vi "Parse-Most_Common_Tile.vi"(10 "Array":T1[](array[typedef])) -> (2 "Tile":T1)   [LabVIEW 2020]
doc: "<B>Description:</B> takes an array of tiles and determines which is the most common and returns that.\n\n<B>Date:</B> 05/2019\n<B>Author:</B> Luke Jarocki, Choose Movement Consulting, LLC"
uses:
  Controls/TileColor.ctl
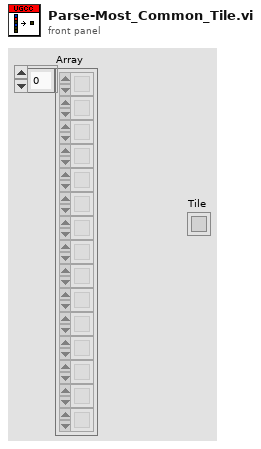
[diagram p1: front panel]
types:
  T1 = typedef "TileColor.ctl" = u16
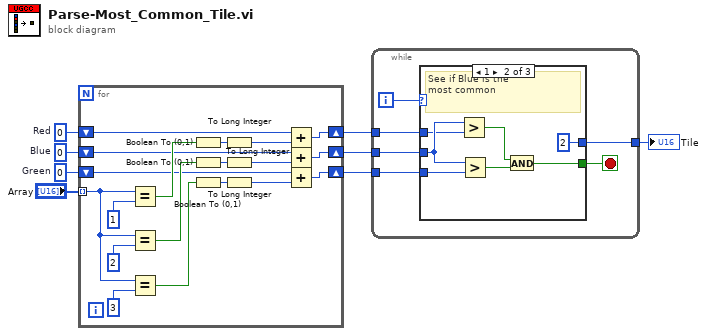
[diagram p0: block diagram]
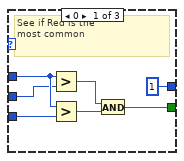
[diagram p2: hidden frame]
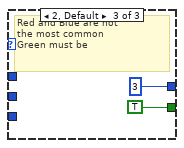
[diagram p3: hidden frame]
diagram:
  w5 = 0  # Green
  w6 = 0  # Blue
  w7 = 0  # Red
  n1 = for {
    tunnel: "Array" -> [w18] mode=indexing
    shift-right: [w24] -> w4
    shift-left: w7 -> [w25]
    shift-right: [w19] -> w3
    shift-left: w6 -> [w20]
    shift-right: [w15] -> w2
    shift-left: w5 -> [w16]
    n2 = Equal?(x=w18, y=T1 1 ("Tile")) -> (x = y?=w26:bool)
    n3 = Equal?(x=w18, y=T1 2 ("Tile")) -> (x = y?=w23:bool)
    n4 = Equal?(x=w18, y=T1 3 ("Tile")) -> (x = y?=w22:bool)
    n5 = Boolean To (0,1)(Boolean=w26) -> (0, 1=w14:i16)
    n6 = Boolean To (0,1)(Boolean=w23) -> (0, 1=w11:i16)
    n7 = Boolean To (0,1)(Boolean=w22) -> (0, 1=w12:i16)
    n8 = To Long Integer(number=w14) -> (32bit integer=w13:i32)
    n9 = To Long Integer(number=w11) -> (32bit integer=w10:i32)
    n10 = To Long Integer(number=w12) -> (32bit integer=w9:i32)
    n11 = Add(x=w25, y=w13) -> (x+y=w24:i32)
    n12 = Add(x=w20, y=w10) -> (x+y=w19:i32)
    n13 = Add(x=w16, y=w9) -> (x+y=w15:i32)
  }
  n14 = while {
    tunnel: w4 -> [w32]
    tunnel: w3 -> [w31]
    tunnel: w2 -> [w30]
    tunnel: [w28] -> w1
    i -> [w33]
    stop <- w29 stop-if-true
    n15 = case shown="1" w33 {
      tunnel: w32 -> [w40 w43 _]
      tunnel: w31 -> [w39 w45 _]
      tunnel: w30 -> [w38 w44 _]
      tunnel: [w35 w42 TRUE] -> w29
      tunnel: [T1 1 ("Tile") T1 2 ("Tile") T1 3 ("Tile")] -> w28
      frame 0 {
        # "See if Red is the\nmost common"
        n16 = Greater?(x=w40, y=w39) -> (0:w37:bool)
        n17 = Greater?(x=w40, y=w38) -> (0:w36:bool)
        n18 = And(x=w37, y=w36) -> (x .and. y?=w35:bool)
      }
      frame 1 {
        # "See if Blue is the\nmost common"
        n19 = Greater?(x=w45, y=w43) -> (0:w47:bool)
        n20 = Greater?(x=w45, y=w44) -> (0:w46:bool)
        n21 = And(x=w47, y=w46) -> (x .and. y?=w42:bool)
      }
      frame 2, Default {
        # "Red and Blue are not\nthe most common\nGreen must be"
      }
    }
  }
  "Tile" <- w1
